vi "IO Nodes Close References.vi"(7 "Project in":refnum<vi>, 8 "error in (no error)":errorcluster, 9 "IO Nodes":refnum<vi>[][](array[refnum]), 10 "Diagram":refnum<vi>, 11 "vi reference":refnum<vi>) -> (0 "error out":errorcluster)   [LabVIEW 2014, in "Initialization and IO Node Scripting.lvlib"]
uses:
  Initialization and IO Node Scripting.lvlib
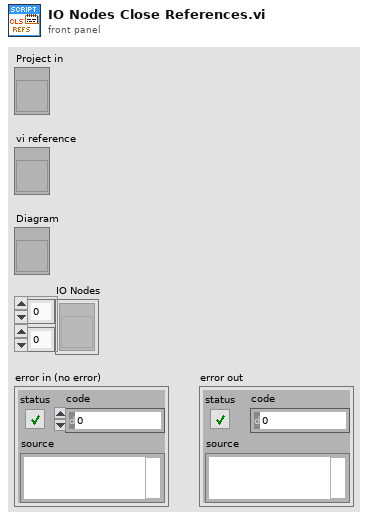
[diagram p1: front panel]
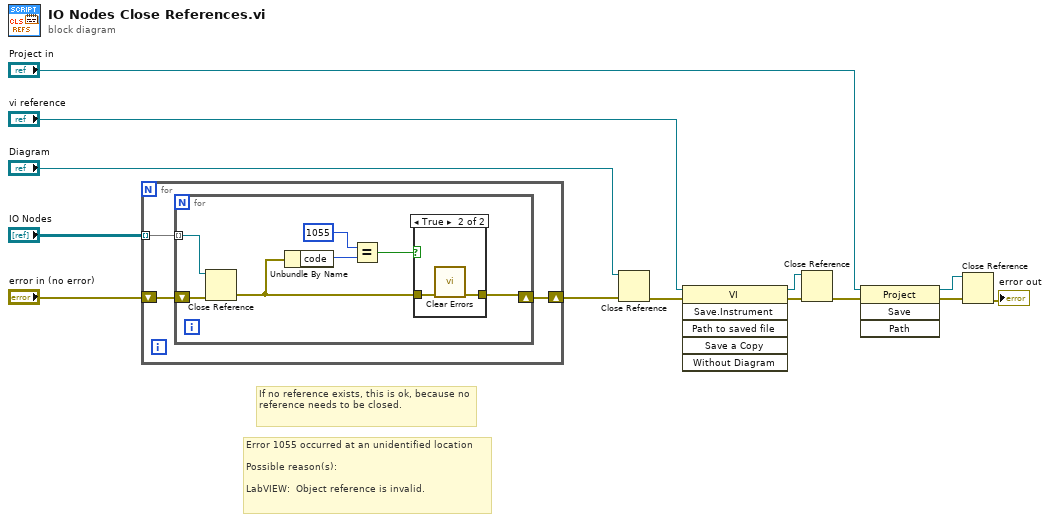
[diagram p0: block diagram]
diagram:
  # "Error 1055 occurred at an unidentified location\n\nPossible reason(s):\n\nLabVIEW:  Object reference is invalid."
  # "If no reference exists, this is ok, because no reference needs to be closed."
  n1 = for {
    shift-right: [w16] -> w3
    shift-left: "error in (no error)" -> [w15]
    tunnel: "IO Nodes" -> [w14] mode=indexing
    n2 = for {
      shift-right: [w21] -> w16
      shift-left: w15 -> [w23]
      tunnel: w14 -> [w22] mode=indexing
      n3 = Close Reference(reference=w22, error in (no error)=w23) -> (error out=w20:errorcluster)
      n4 = Unbundle By Name(w20) -> ("code"=w19:i32)
      n5 = Equal?(x=1055, y=w19) -> (x = y?=w18:bool)
      n6 = case shown="True" w18 {
        tunnel: w20 -> [w24 w26]
        tunnel: [w24 w25] -> w21
        frame False {
        }
        frame True {
          n7 = call <vilib>:"Clear Errors.vi"("error in (no error)"=w26) -> ("error out"=w25:errorcluster)  [unwired: 5 in, 1 out]
        }
      }
    }
  }
  n8 = Close Reference(reference="Diagram", error in (no error)=w3) -> (error out=w5:errorcluster)
  n9 = invoke class="VI" method="Save.Instrument"(reference="vi reference", error in=w5) -> (reference out=w8:refnum<vi>, error out=w6:errorcluster)  [unwired: 4 in, 4 out]
  n10 = Close Reference(reference=w8, error in (no error)=w6) -> (error out=w11:errorcluster)
  n11 = invoke class="Project" method="Save"(reference="Project in", error in=w11) -> (reference out=w10:refnum<vi>, error out=w9:errorcluster)  [unwired: 2 in, 2 out]
  n12 = Close Reference(reference=w10, error in (no error)=w9) -> (error out=→"error out":errorcluster)
